vi "Find Furthest Node.vi"(10 "String in":string, 11 "Map in":map{string, cluster{string[], u64, bool}}(c390)) -> (2 "String out":string, 3 "Map out":map{string, cluster{string[], u64, bool}}(c390))   [LabVIEW 2023, in "d25.lvlib"]
uses:
  d25.lvlib
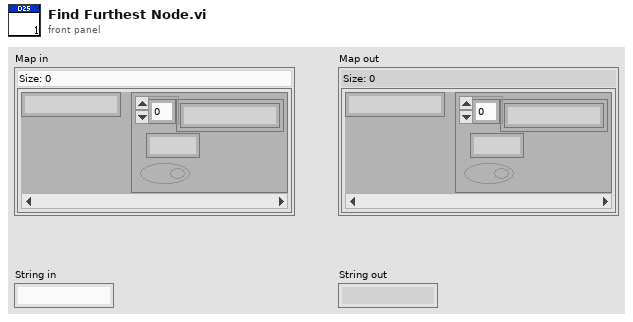
[diagram p1: front panel]
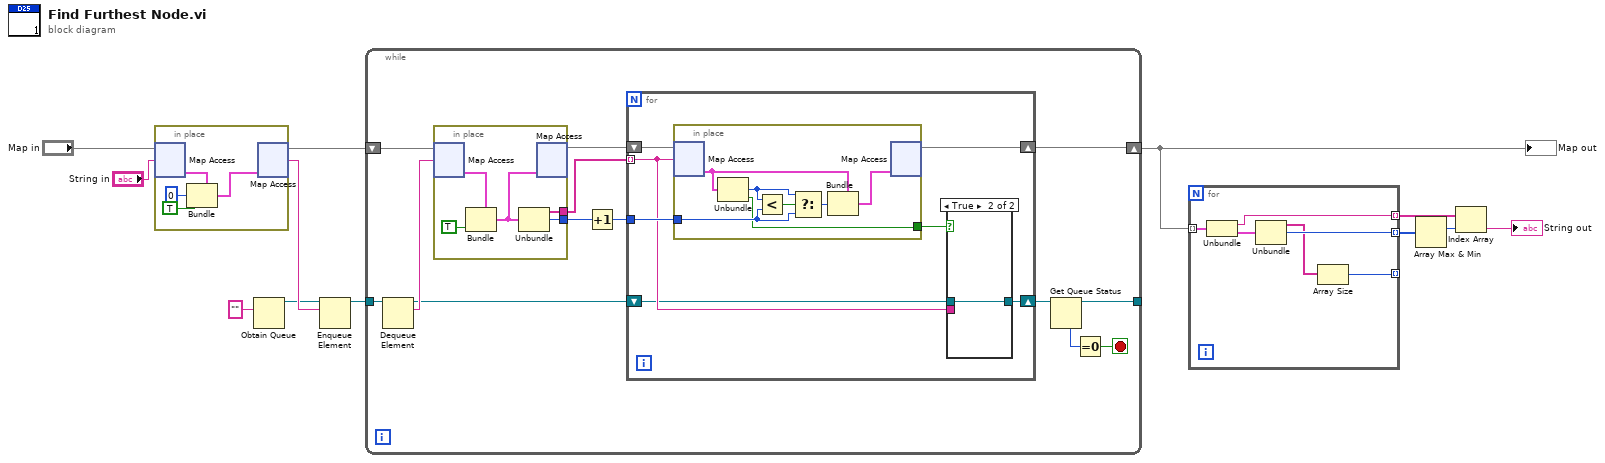
[diagram p0: block diagram]
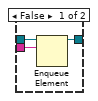
[diagram p2: hidden frame]
diagram:
  n1 = in-place {
    n2 = in-place-map #1("Map in", "String in") -> (w16:cluster{string[], u64, bool})  [unwired: 1 in, 1 out]
    n3 = Bundle(cluster=w16, u64 0, TRUE) -> (w13:cluster{string[], u64, bool})  [unwired: 1 in]
    n4 = in-place-map #1(w13) -> (w3:map{string, cluster{string[], u64, bool}}, w7:string)  [unwired: 1 in, 1 out]
  }
  n5 = Obtain Queue(element data type="" ("search string/char (-)")) -> (queue out=w4:refnum<queue>)  [unwired: 4 in, 2 out]
  n6 = Enqueue Element(queue=w4, element=w7) -> (queue out=w6:refnum<queue>)  [unwired: 2 in, 2 out]
  n7 = while {
    shift-right: [w25] -> w8
    shift-left: w3 -> [w28]
    tunnel: w6 -> [w29]
    tunnel: [w19] -> _
    stop <- w17 stop-if-true
    n8 = Dequeue Element(queue=w29) -> (queue out=w21:refnum<queue>, element=w27:string)  [unwired: 2 in, 2 out]
    n9 = in-place {
      in-place-border: [w49] -> w24
      in-place-border: [w48] -> w23
      n10 = in-place-map #2(w28, w27) -> (w52:cluster{string[], u64, bool})  [unwired: 1 in, 1 out]
      n11 = Bundle(cluster=w52, TRUE) -> (w50:cluster{string[], u64, bool})  [unwired: 2 in]
      n12 = Unbundle(w50) -> (w49:string[], w48:u64)  [unwired: 1 out]
      n13 = in-place-map #2(w50) -> (w26:map{string, cluster{string[], u64, bool}})  [unwired: 1 in, 2 out]
    }
    n14 = Increment(x=w23) -> (x+1=w22:u64)
    n15 = for {
      shift-right: [w35] -> w25
      shift-left: w26 -> [w36]
      tunnel: w24 -> [w33] mode=indexing
      tunnel: w22 -> [w34]
      shift-right: [w30] -> w20
      shift-left: w21 -> [w32]
      n16 = in-place {
        in-place-border: w34 -> [w42]
        in-place-border: [w41] -> w31
        n17 = in-place-map #3(w36, w33) -> (w46:cluster{string[], u64, bool})  [unwired: 1 in, 1 out]
        n18 = Unbundle(w46) -> (w44:u64, w41:bool)  [unwired: 1 out]
        n19 = Less?(x=w44, y=w42) -> (x < y?=w45:bool)
        n20 = Select(t=w44, s=w45, f=w42) -> (s? t:f=w43:u64)
        n21 = Bundle(cluster=w46, w43) -> (w47:cluster{string[], u64, bool})  [unwired: 2 in]
        n22 = in-place-map #3(w47) -> (w35:map{string, cluster{string[], u64, bool}})  [unwired: 1 in, 2 out]
      }
      n23 = case shown="True" w31 {
        tunnel: w33 -> [w39 _]
        tunnel: w32 -> [w38 w40]
        tunnel: [w37 w40] -> w30
        frame False {
          n24 = Enqueue Element(queue=w38, element=w39) -> (queue out=w37:refnum<queue>)  [unwired: 2 in, 2 out]
        }
        frame True {
        }
      }
    }
    n25 = Get Queue Status(queue=w20) -> (queue out=w19:refnum<queue>, # elements in queue=w18:i32)  [unwired: 2 in, 6 out]
    n26 = Equal To 0?(x=w18) -> (x = 0?=w17:bool)
  }
  "Map out" <- w8
  n27 = for {
    tunnel: w8 -> [w58] mode=indexing
    tunnel: [w56] -> w9 mode=indexing
    tunnel: [w55] -> w12 mode=indexing
    tunnel: [w53] -> _ mode=indexing
    n28 = Unbundle(w58) -> (w55:string, w57:cluster{string[], u64, bool})
    n29 = Unbundle(w57) -> (w54:string[], w56:u64)  [unwired: 1 out]
    n30 = Array Size(array=w54) -> (size(s)=w53:i32)
  }
  n31 = Array Max & Min(array=w9) -> (max index (indices)=w10:i32)  [unwired: 3 out]
  n32 = Index Array(array=w12, index=w10) -> (element=→"String out":string)
